vi "temp_rods.vi"() -> ()   [LabVIEW 2009]
uses:
  <vilib>/Math Plots/3D Math Plots/3D Contour/3D Contour XCtrl/3D Contour.xctl
  <vilib>/Utility/file.llb/Write To Spreadsheet File (DBL).vi
  <vilib>/Math Plots/3D Math Plots/3D Contour/3D Contour Datatype/Public/Plot Helper (Vector).vi
  <vilib>/Math Plots/3D Math Plots/3D Contour/3D Contour Datatype/3D Contour Datatype.lvclass
panel:
  out "Temps":dbl[](array[numeric])
  in  "Plot 3D?":bool
  out "T(t,x)":refnum<class "3D Plot Datatype.lvclass">[](xcontrol)
  in  "Clear Data":bool
  in  "Record Data":bool
  in  "CSV Save Path":path
  in  "Save Data To CSV?":bool
  in  "Stop VI":bool
  out "Temp Plot":cluster{"Range":i64[], "Array":dbl[]}(graph)
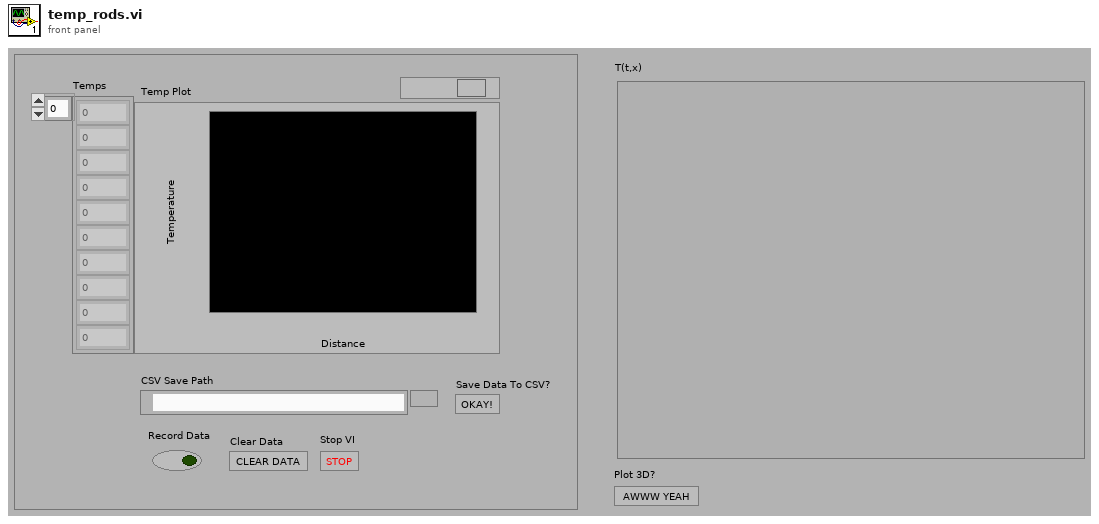
[diagram p1: front panel]
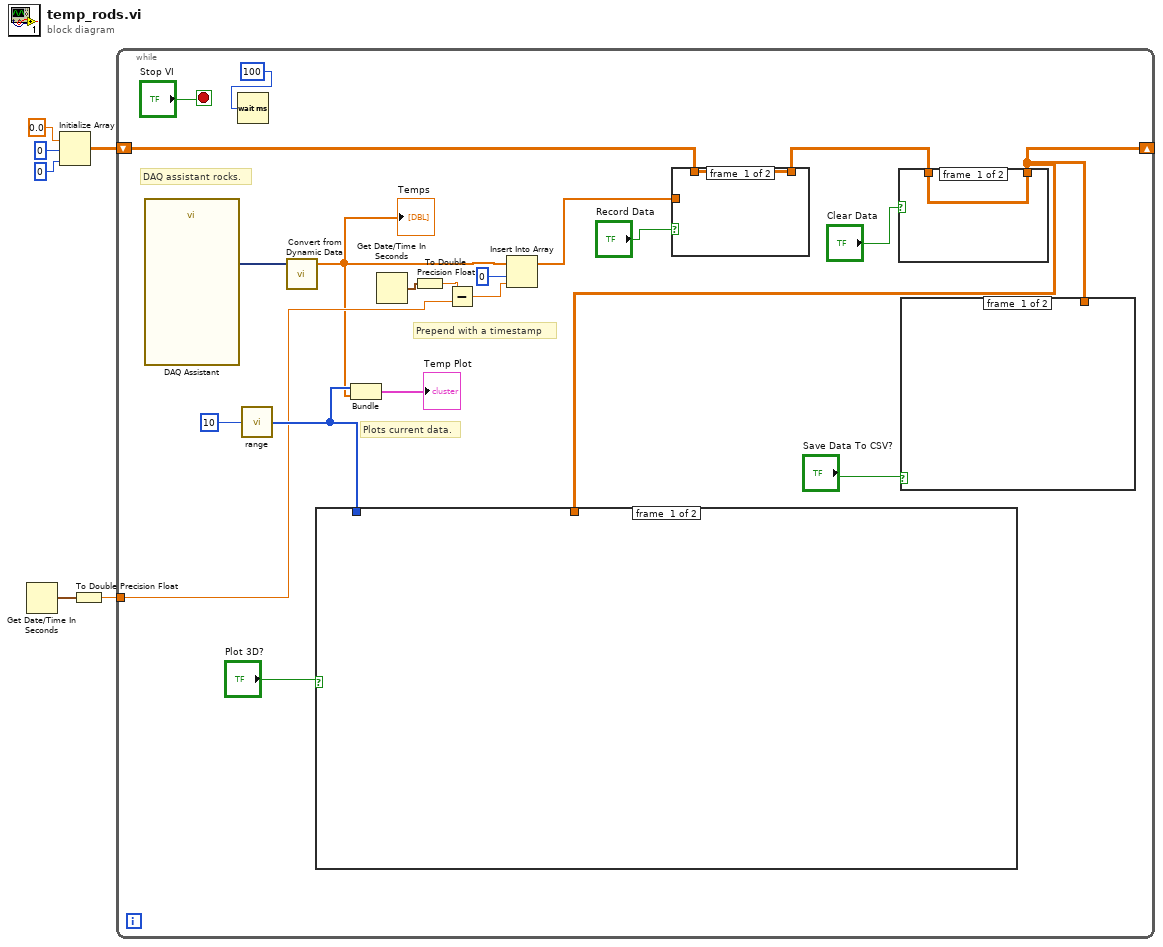
[diagram p0: block diagram]
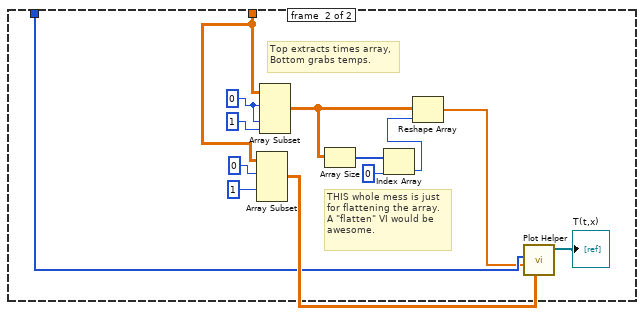
[diagram p2: hidden frame]
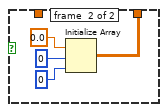
[diagram p3: hidden frame]
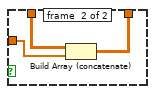
[diagram p4: hidden frame]
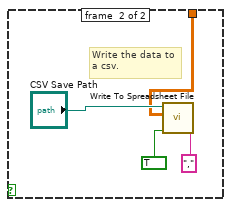
[diagram p5: hidden frame]
diagram:
  n1 = Get Date/Time In Seconds() -> (seconds since 1Jan1904=w1:timestamp)
  n2 = Initialize Array(0.0, 0, 0) -> (w5:dbl[][])
  n3 = To Double Precision Float(number=w1) -> (double precision float=w2:dbl)
  n4 = while {
    shift-right: [w7] -> _
    shift-left: w5 -> [w19]
    tunnel: w2 -> [w13]
    stop <- "Stop VI" stop-if-true
    # "DAQ assistant rocks."
    # "Plots current data."
    # "Prepend with a timestamp"
    n5 = call "DAQ Assistant"() -> ("data"=w24:dynamicdata)  [unwired: 17 in, 2 out]
    n6 = Wait (ms)(milliseconds to wait=100) -> ()  [unwired: 1 out]
    n7 = call "range.vi"("to"=10) -> ("Range"=w15:i64[])  [unwired: 4 in]
    n8 = call "Convert from Dynamic Data"("Dynamic Data Type"=w24) -> ("Array"=w8:dbl[])  [unwired: 3 in]
    "Temps" <- w8
    n9 = Bundle("Range"=w15, "Array"=w8) -> (→"Temp Plot":cluster{"Range":i64[], "Array":dbl[]})  [unwired: 1 in]
    n10 = Get Date/Time In Seconds() -> (seconds since 1Jan1904=w11:timestamp)
    n11 = To Double Precision Float(number=w11) -> (double precision float=w10:dbl)
    n12 = Subtract(x=w10, y=w13) -> (x-y=w12:dbl)
    n13 = Insert Into Array(array=w8, index=0, new element=w12) -> (w20:dbl[])
    n14 = case shown="True" "Record Data" {
      tunnel: w20 -> [_ w48]
      tunnel: w19 -> [w45 w47]
      tunnel: [w45 w46] -> w16
      frame #0 {
      }
      frame #1 {
        n15 = Build Array (concatenate)(w47, w48) -> (w46:dbl[][])
      }
    }
    n16 = case shown="True" "Clear Data" {
      tunnel: w16 -> [w40 _]
      tunnel: [w40 w41] -> w7
      frame #0 {
      }
      frame #1 {
        n17 = Initialize Array(0.0, 0, 0) -> (w41:dbl[][])
      }
    }
    n18 = case shown="True" "Plot 3D?" {
      tunnel: w7 -> [_ w39]
      tunnel: w15 -> [_ w28]
      frame #0 {
      }
      frame #1 {
        w36 = 0
        # "THIS whole mess is just\nfor flattening the array.\nA \"flatten\" VI would be\nawesome."
        # "Top extracts times array,\nBottom grabs temps."
        n19 = Array Subset(array=w39, index (row)=0, index (col)=1) -> (w30:dbl[][])  [unwired: 2 in]
        n20 = Array Subset(array=w39, index (row)=w36, index (col)=w36, length (col)=1) -> (w34:dbl[][])  [unwired: 1 in]
        n21 = Array Size(array=w34) -> (size(s)=w38:i32[])
        n22 = Index Array(array=w38, index=0) -> (element=w35:i32)
        n23 = Reshape Array(w34, w35) -> (w27:dbl[])
        n24 = call-poly <vilib>:"Plot Helper.vi"("z matrix"=w30, "y vector"=w27, "x vector"=w28) -> ("3D Plot lvclass Array out"=→"T(t,x)":refnum<class "3D Plot Datatype.lvclass">[])  [unwired: 3 in, 5 out]
      }
    }
    n25 = case shown="True" "Save Data To CSV?" {
      tunnel: w7 -> [_ w49]
      frame #0 {
      }
      frame #1 {
        # "Write the data to\na csv."
        n26 = call-poly <vilib>:"Write To Spreadsheet File.vi"("delimiter (\\t)"=",", "append to file? (new file:F)"=TRUE, "2D data"=w49, "file path (dialog if empty)"="CSV Save Path") -> ()  [unwired: 4 in, 1 out]
      }
    }
  }
